vi "power_meter.vi"() -> ()   [LabVIEW 2016]
panel:
  out "Voltage (V)":dbl
  in  "stop":bool
  out "Power (mW)":dbl
  in  "PD Gain (V/mW)":dbl
  out "Waveform Chart":dynamicdata(graph)
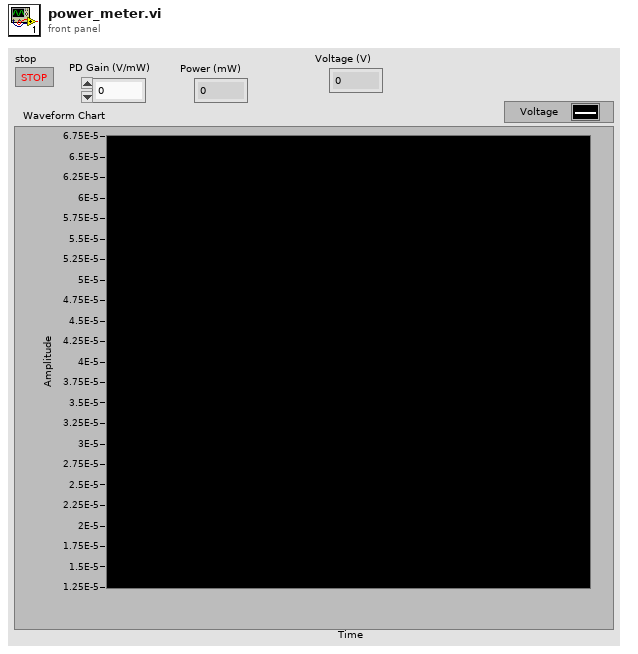
[diagram p1: front panel]
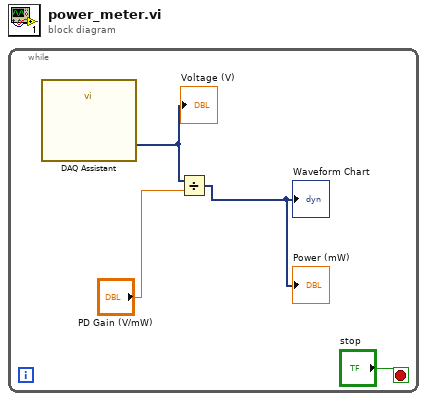
[diagram p0: block diagram]
diagram:
  n1 = while {
    stop <- "stop" stop-if-true
    n2 = call "DAQ Assistant"() -> ("data"=w1:dynamicdata)  [unwired: 17 in, 2 out]
    "Voltage (V)" <- w1
    n3 = Divide(x=w1, y="PD Gain (V/mW)") -> (x/y=→"Waveform Chart" →"Power (mW)":dynamicdata)
  }
